vi "loadImageAndConvert.vi"(8 "error in (no error)":errorcluster, 10 "name or relative path":string) -> (0 "error out":errorcluster, 2 ".NET object":refnum<k24>)   [LabVIEW 2014, in "DataGridView.lvclass"]
uses:
  DataGridView.lvclass
  System.Drawing
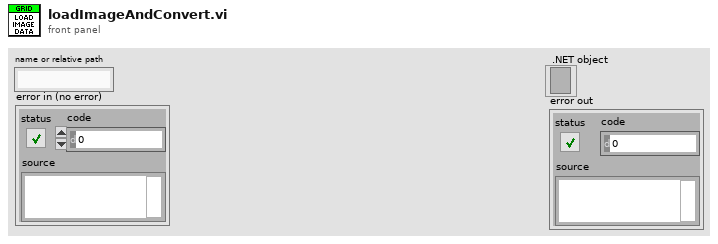
[diagram p1: front panel]
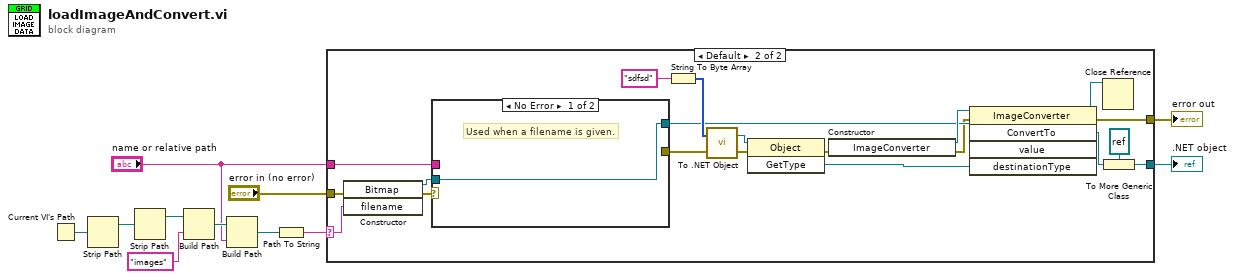
[diagram p0: block diagram]
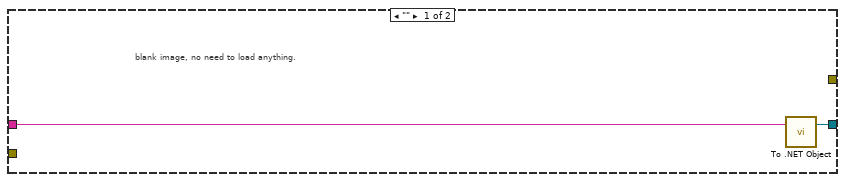
[diagram p2: hidden frame]
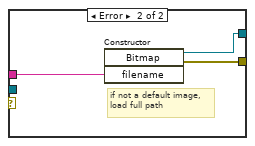
[diagram p3: hidden frame]
diagram:
  n1 = Current VI's Path() -> (path=w10:path)
  n2 = Strip Path(path=w10) -> (stripped path=w9:path)  [unwired: 1 out]
  n3 = Strip Path(path=w9) -> (stripped path=w7:path)  [unwired: 1 out]
  n4 = Build Path(base path=w7, name or relative path="images") -> (appended path=w6:path)
  n5 = Build Path(base path=w6, name or relative path="name or relative path") -> (appended path=w5:path)
  n6 = Path To String(path=w5) -> (string=w11:string)
  n7 = case shown="Default" w11 {
    selector: w11 -> [_ w33]
    tunnel: "name or relative path" -> [w13 w31]
    tunnel: [w12 w28] -> w3
    tunnel: "error in (no error)" -> [_ w16]
    tunnel: [_ w15] -> w1
    frame "" {
      # "blank image, no need to load anything."
      n8 = call <vilib>:"To .NET Object.vi"("anything"=w13) -> (".NET object"=w12:refnum<k24>)  [unwired: 1 in, 1 out]
    }
    frame Default {
      n9 = constructor class="Bitmap"(error in=w16, "filename"=w33) -> (reference out=w30:refnum<k24>, error out=w32:errorcluster)  [unwired: 2 in, 2 out]
      n10 = case shown="No Error" w32 {
        tunnel: w31 -> [_ w37]
        tunnel: [w34 w36] -> w23
        tunnel: w30 -> [w34 _]
        tunnel: [_ w35] -> w20
        frame No Error {
          # "Used when a filename is given."
        }
        frame Error {
          # "if not a default image,\nload full path"
          n11 = constructor class="Bitmap"("filename"=w37) -> (reference out=w36:refnum<k24>, error out=w35:errorcluster)  [unwired: 3 in, 2 out]
        }
      }
      n12 = String To Byte Array(string="sdfsd") -> (unsigned byte array=w25:u8[])
      n13 = call <vilib>:"To .NET Object.vi"("error in (no error)"=w20, "anything"=w25) -> ("error out"=w19:errorcluster, ".NET object"=w26:refnum<k24>)
      n14 = invoke class="Object" method="GetType"(reference=w26, error in=w19) -> (error out=w18:errorcluster, "GetType"=w27:refnum<k24>)  [unwired: 1 in, 1 out]
      n15 = constructor class="ImageConverter"(error in=w18) -> (reference out=w24:refnum<k24>, error out=w17:errorcluster)  [unwired: 2 in, 1 out]
      n16 = invoke class="ImageConverter" method="ConvertTo"(reference=w24, error in=w17, "value"=w23, "destinationType"=w27) -> (reference out=w14:refnum<k24>, error out=w15:errorcluster, "ConvertTo"=w22:refnum<k24>)  [unwired: 1 in, 2 out]
      n17 = Close Reference(reference=w14) -> ()  [unwired: 1 in, 1 out]
      n18 = To More Generic Class(target class=refnum<k24> refnum (".NET object"), reference=w22) -> (generic class reference=w28:refnum<k24>)
    }
  }
  ".NET object" <- w3
  "error out" <- w1
